vi "To Start and Stop.vi"   [LabVIEW 2009]
doc: "Takes two numbers (can have units) that indicate the average (\"center\") and difference (\"span\") of two numbers and returns the beginning and end of the range."
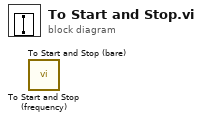
[diagram p0: block diagram]
diagram:
  n1 = call "To Start and Stop (frequency).vi"() -> ()  [unwired: 6 in, 2 out]
  n2 = call "To Start and Stop (bare).vi"() -> ()  [unwired: 6 in, 2 out]
